vi "BASE_Create Login.vi"(6 "Error In":errorcluster, 8 "Password":string, 9 "User Name":string(combo)) -> (0 "error out":errorcluster)   [LabVIEW 2017]
uses:
  <vilib>/Utility/config.llb/Write Key (String).vi
  <vilib>/Utility/config.llb/Write Key (I32).vi
  <vilib>/Utility/config.llb/NI_LVConfig.lvlib
panel:
  in  "Level":u16(ring) items=["", "Operator", "Superviser", "Admin"]
  in  "Delete":bool
  in  "Exit":bool
  in  "Create":bool
  # "CREATE LOGIN"
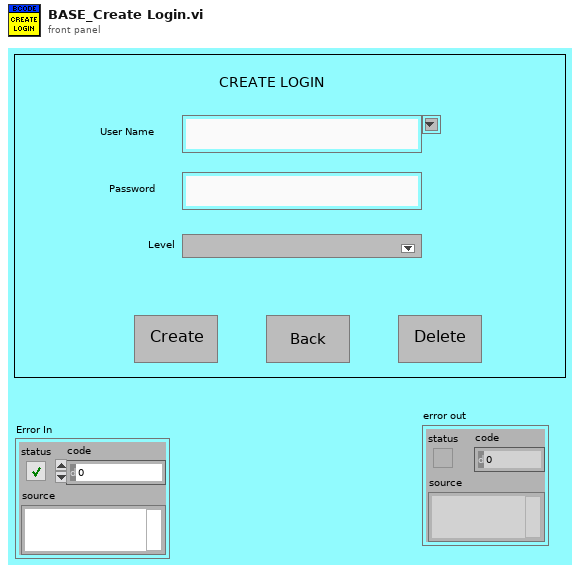
[diagram p1: front panel]
types:
  T1 = enum32{"invalid app kind", "Development System", "Run Time System", "Student Edition", "Embedded LabVIEW", "Evaluation", "Custom"}
  T2 = typedef "NI_LVConfig.lvlib/Config Data RefNum.ctl" = refnum<k1>
  T3 = enum32{"Invalid", "Standard", "Closed", "Hidden", "Minimized", "Maximized"}
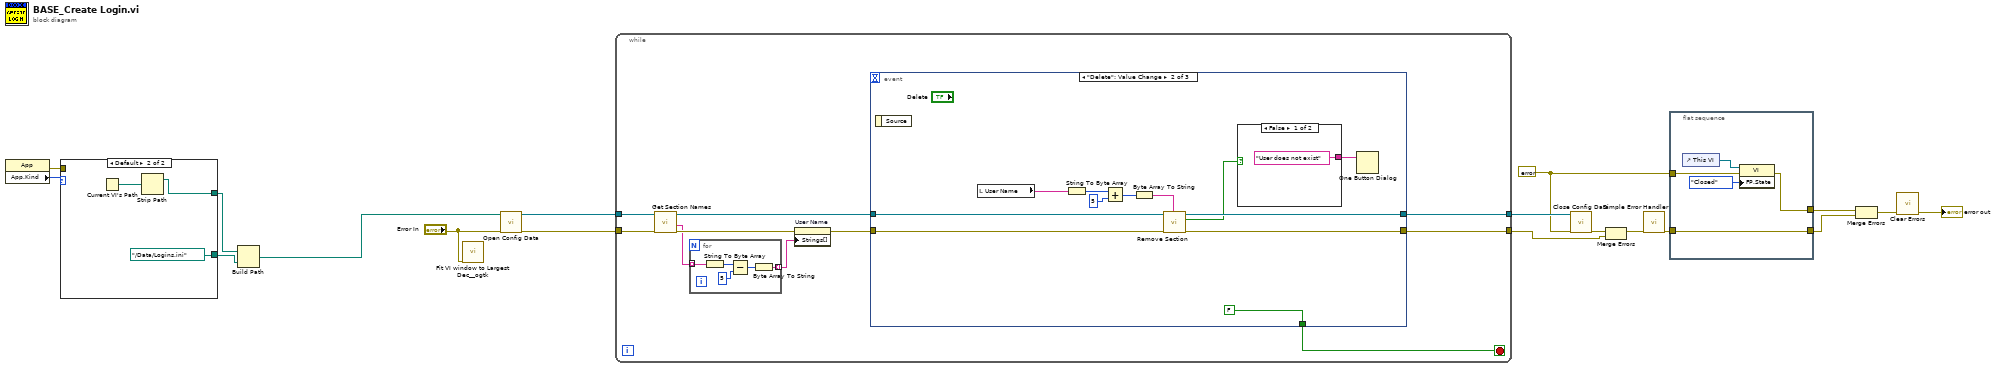
[diagram p0: block diagram]
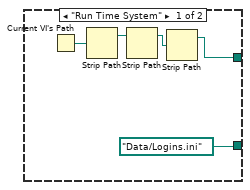
[diagram p2: hidden frame]
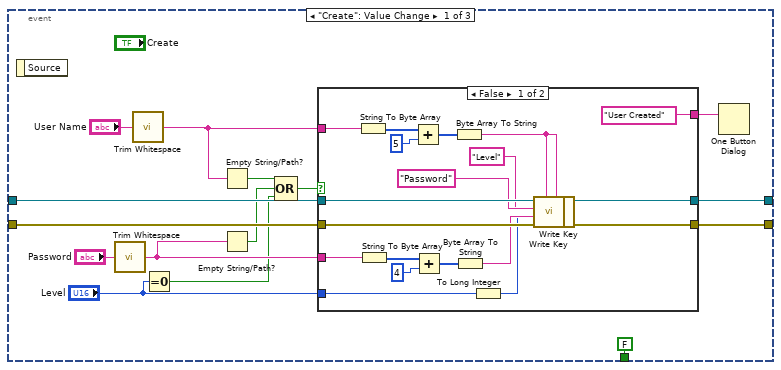
[diagram p3: hidden frame]
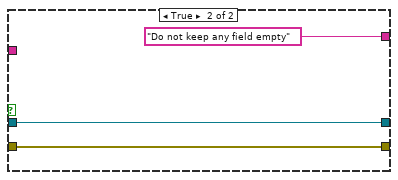
[diagram p4: hidden frame]
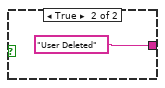
[diagram p5: hidden frame]
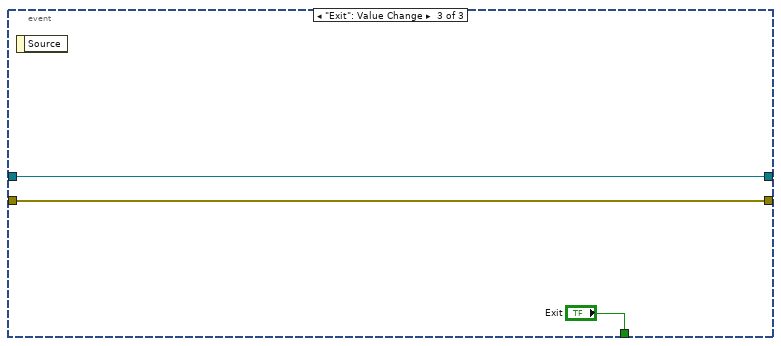
[diagram p6: hidden frame]
diagram:
  w16 = errorcluster {"status"=FALSE, "code"=0, "source"=""} ("error in (no error)")
  n1 = property class="App"() -> (error out=w3:errorcluster, "App.Kind"=w5:T1)  [unwired: 2 in, 1 out]
  n2 = case shown="Default" w5 {
    tunnel: [w20 w25] -> w2
    tunnel: [path "Data/Logins.ini" ("path") path "../Data/Logins.ini" ("path")] -> w4
    tunnel: w3 -> [_ _]
    frame "Run Time System" {
      n3 = Current VI's Path() -> (path=w23:path)
      n4 = Strip Path(path=w23) -> (stripped path=w22:path)  [unwired: 1 out]
      n5 = Strip Path(path=w22) -> (stripped path=w21:path)  [unwired: 1 out]
      n6 = Strip Path(path=w21) -> (stripped path=w20:path)  [unwired: 1 out]
    }
    frame Default {
      n7 = Current VI's Path() -> (path=w26:path)
      n8 = Strip Path(path=w26) -> (stripped path=w25:path)  [unwired: 1 out]
    }
  }
  n9 = Build Path(base path=w2, name or relative path=w4) -> (appended path=w1:path)
  n10 = call <userlib>:"Fit VI window to Largest Dec__ogtk.vi"("error in (no error)"="Error In") -> ()  [unwired: 5 in, 2 out]
  n11 = call <vilib>:"Open Config Data.vi"("error in (no error)"="Error In", "configuration file path"=w1) -> ("error out"=w10:errorcluster, "refnum"=w9:T2)  [unwired: 7 in, 1 out]
  n12 = while {
    tunnel: [w36] -> w7
    tunnel: [w35] -> w18
    tunnel: w10 -> [w33]
    tunnel: w9 -> [w32]
    stop <- w34 stop-if-true
    n13 = call <vilib>:"Get Section Names.vi"("error in (no error)"=w33, "refnum"=w32) -> ("error out"=w30:errorcluster, "section names"=w28:string[], "refnum out"=w31:T2)  [unwired: 7 in]
    n14 = for {
      tunnel: w28 -> [w97] mode=indexing
      tunnel: [w93] -> w27 mode=indexing
      n15 = String To Byte Array(string=w97) -> (unsigned byte array=w96:u8[])
      n16 = Subtract(x=w96, y=u8 5) -> (x-y=w94:u8[])
      n17 = Byte Array To String(unsigned byte array=w94) -> (string=w93:string)
    }
    n18 = property on="User Name" class="CmbBox"(error in=w30, "Strings[]"=w27) -> (error out=w29:errorcluster)  [unwired: 1 in, 1 out]
    n19 = event shown="[1] \"Delete\": Value Change" {
      selector: _ -> [_ _ _]
      dyn-events: _ -> [_ _ _]
      timeout: _ -> [_ _ _]
      tunnel: w31 -> [w51 w87 w91]
      tunnel: w29 -> [w50 w86 w90]
      tunnel: [w47 w84 w90] -> w36
      tunnel: [w48 w85 w91] -> w35
      tunnel: [FALSE ("Exit") FALSE ("Exit") "Exit"] -> w34
      event "Create": Value Change {
        n20 = event-data() -> ()  [unwired: 1 in, 1 out]
        n21 = call <vilib>:"Trim Whitespace.vi"("string"="Password") -> ("trimmed string"=w40:string)  [unwired: 1 in]
        n22 = call <vilib>:"Trim Whitespace.vi"("string"="User Name") -> ("trimmed string"=w41:string)  [unwired: 1 in]
        n23 = Equal To 0?(x="Level") -> (x = 0?=w38:bool)
        n24 = Empty String/Path?(string/path=w41) -> (empty?=w46:bool)
        n25 = Empty String/Path?(string/path=w40) -> (empty?=w45:bool)
        n26 = Compound Arithmetic op=OR(w46, w45, w38) -> (w44:bool)
        n27 = case shown="False" w44 {
          tunnel: w51 -> [w72 w75]
          tunnel: w50 -> [w71 w74]
          tunnel: [w57 w75] -> w48
          tunnel: [w59 w74] -> w47
          tunnel: w41 -> [w61 _]
          tunnel: w40 -> [w69 _]
          tunnel: "Level" -> [w53 _]
          tunnel: ["User Created" ("message") "Do not keep any field empty" ("message")] -> w37
          frame False {
            n28 = String To Byte Array(string=w61) -> (unsigned byte array=w62:u8[])
            n29 = String To Byte Array(string=w69) -> (unsigned byte array=w68:u8[])
            n30 = Add(x=w62, y=u8 5) -> (x+y=w64:u8[])
            n31 = Add(x=w68, y=u8 4) -> (x+y=w66:u8[])
            n32 = Byte Array To String(unsigned byte array=w64) -> (string=w56:string)
            n33 = Byte Array To String(unsigned byte array=w66) -> (string=w65:string)
            n34 = To Long Integer(number=w53) -> (32bit integer=w54:i32)
            n35 = call-poly <vilib>:"Write Key.vi"("section"=w56, "error in (no error)"=w71, "value"=w65, "key"="Password", "refnum"=w72) -> ("error out"=w60:errorcluster, "refnum out"=w58:T2)  [unwired: 4 in, 1 out]
            n36 = call-poly <vilib>:"Write Key.vi"("section"=w56, "error in (no error)"=w60, "value"=w54, "key"="Level", "refnum"=w58) -> ("error out"=w59:errorcluster, "refnum out"=w57:T2)  [unwired: 4 in, 1 out]
          }
          frame True {
          }
        }
        n37 = One Button Dialog(message=w37) -> ()  [unwired: 1 in, 1 out]
      }
      event "Delete": Value Change {
        n38 = event-data() -> ()  [unwired: 1 in, 1 out]
        n39 = local read "User Name"() -> (w79:string)
        n40 = String To Byte Array(string=w79) -> (unsigned byte array=w80:u8[])
        n41 = Add(x=w80, y=u8 5) -> (x+y=w82:u8[])
        n42 = Byte Array To String(unsigned byte array=w82) -> (string=w78:string)
        n43 = call <vilib>:"Remove Section.vi"("section"=w78, "error in (no error)"=w86, "refnum"=w87) -> ("error out"=w84:errorcluster, "section exists?"=w77:bool, "refnum out"=w85:T2)  [unwired: 6 in]
        n44 = case shown="False" w77 {
          tunnel: ["User does not exist" ("message") "User Deleted" ("message")] -> w76
          frame False {
          }
          frame True {
          }
        }
        n45 = One Button Dialog(message=w76) -> ()  [unwired: 1 in, 1 out]
      }
      event "Exit": Value Change {
        n46 = event-data() -> ()  [unwired: 1 in, 1 out]
      }
    }
  }
  n47 = call <vilib>:"Close Config Data.vi"("error in (no error)"=w16, "refnum"=w18) -> ("error out"=w17:errorcluster)  [unwired: 8 in, 1 out]
  n48 = Merge Errors(w17, w7) -> (w8:errorcluster)
  n49 = call <vilib>:"Simple Error Handler.vi"("error in (no error)"=w8) -> ("error out"=w11:errorcluster)  [unwired: 4 in, 4 out]
  n50 = flat-sequence {
    tunnel: w16 -> [w100]
    tunnel: [w99] -> w15
    tunnel: [w98] -> w12
    tunnel: w11 -> [w98]
    frame #0 {
      n51 = control-ref of="This VI"() -> (w102:refnum<vi>)
      n52 = property class="VI"(reference=w102, error in=w100, "FP.State"=T3."Closed" ("Front Panel Window:State")) -> (error out=w99:errorcluster)  [unwired: 1 out]
    }
  }
  n53 = Merge Errors(w15, w12) -> (w14:errorcluster)
  n54 = call <vilib>:"Clear Errors.vi"("error in (no error)"=w14) -> ("error out"=→"error out":errorcluster)  [unwired: 5 in, 1 out]
